vi "SparkMAXCommandPower.vi"(0 "Device Reference (in)":T2, 5 "Output Mode":T1(ring), 7 "Control Mode":enum16{"Safety", "Power"}(ring), 9 "Power or Testing Power":dbl, 11 "Error (in)":errorcluster) -> ()   [LabVIEW 2023]
doc: "Wrapper for commanding the power of a Talon FX motor controller. Supports voltage and safety interlock. Also supports the standard actuator testing interface and and the only sending new values on change."
uses:
  <vilib>/Rock Robotics/WPI/MotorControl/WPI_MotorControlDeviceRef.ctl
  <vilib>/Rock Robotics/WPI/MotorControl/WPI_MotorControlType.ctl
  <vilib>/Rock Robotics/SystemInterfaces/DIO/FPGA_DIOPWMChannel.ctl
  <vilib>/Rock Robotics/WPI/PWM/WPI_PWMDeadband.ctl
  <vilib>/Rock Robotics/SystemInterfaces/DIO/FPGA_DIOChannel.ctl
  <vilib>/Rock Robotics/WPI/ThirdParty/REV Robotics/REVLib/Typedef/Spark MAX Control Type.ctl
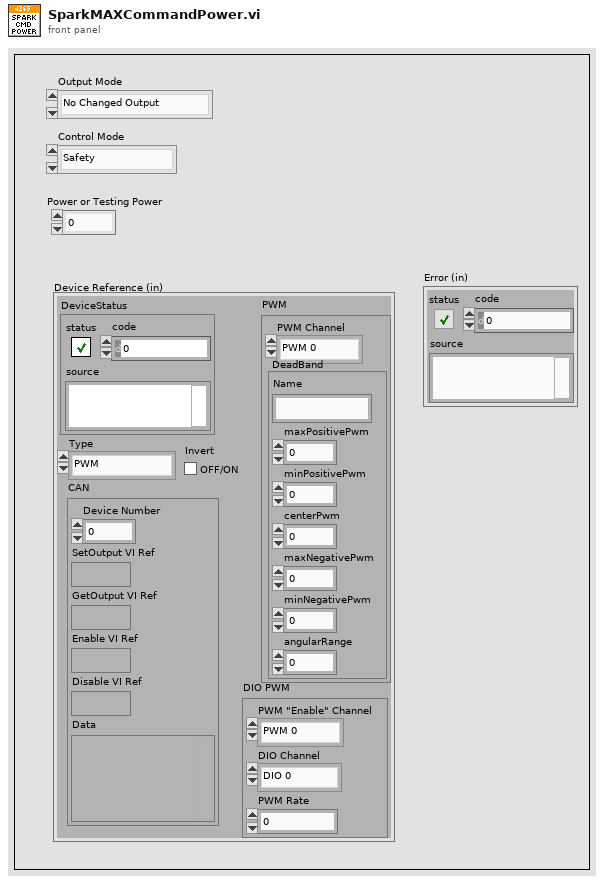
[diagram p1: front panel]
types:
  T1 = enum16{"No Changed Output", "New Normal Output", "New Testing Output"}
  T2 = typedef "WPI_MotorControlDeviceRef.ctl" = cluster{"DeviceStatus":errorcluster, "Type":T3, "PWM":cluster{"PWM Channel":T4, "DeadBand":T5}, "CAN":cluster{"Device Number":u8, "SetOutput VI Ref":variant, "GetOutput VI Ref":variant, "Enable VI Ref":variant, "Disable VI Ref":variant, "Data":variant}, "Invert":bool, "DIO PWM":cluster{"PWM \"Enable\" Channel":T4, "DIOChannel":T6, "PWM Rate":dbl}}
  T3 = typedef "WPI_MotorControlType.ctl" = enum16{"PWM", "CAN", "DIO PWM"}
  T4 = typedef "FPGA_DIOPWMChannel.ctl" = enum8{"PWM 0", "PWM 1", "PWM 2", "PWM 3", "PWM 4", "PWM 5", "PWM 6", "PWM 7", "PWM 8", "PWM 9", "PWM MXP 0", "PWM MXP 1", "PWM MXP 2", "PWM MXP 3", "PWM MXP 4", "PWM MXP 5", "PWM MXP 6", "PWM MXP 7", "PWM MXP 8", "PWM MXP 9", "Invalid"}
  T5 = typedef "WPI_PWMDeadband.ctl" = cluster{"Name":string, "maxPositivePwm":i32, "minPositivePwm":i32, "centerPwm":i32, "maxNegativePwm":i32, "minNegativePwm":i32, "angularRange":u16}
  T6 = typedef "FPGA_DIOChannel.ctl" = enum8{"DIO 0", "DIO 1", "DIO 2", "DIO 3", "DIO 4", "DIO 5", "DIO 6", "DIO 7", "DIO 8", "DIO 9", "DIO MXP 0", "DIO MXP 1", "DIO MXP 2", "DIO MXP 3", "DIO MXP 4", "DIO MXP 5", "DIO MXP 6", "DIO MXP 7", "DIO MXP 8", "DIO MXP 9", "DIO MXP 10", "DIO MXP 11", "DIO MXP 12", "DIO MXP 13", "DIO MXP 14", "DIO MXP 15", "SPI Port CS1", "SPI Port CS2", "SPI Port CS3", "SPI Port MISO", "SPI Port MOSI", "Invalid"}
  T7 = typedef "Spark MAX Control Type.ctl" = enum16{"Percent VBus", "Voltage", "Velocity", "Position", "Smart Motion", "Current", "Smart Velocity"}
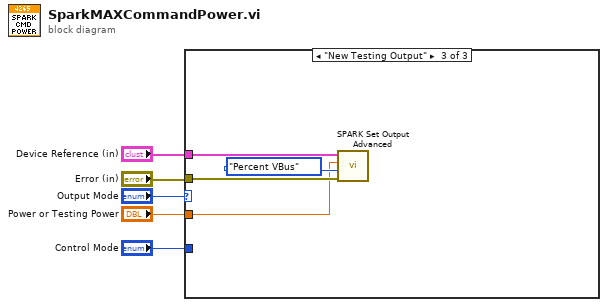
[diagram p0: block diagram]
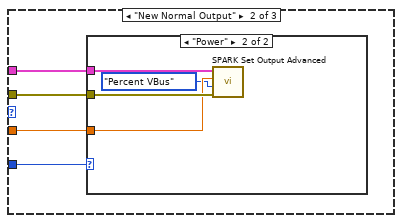
[diagram p3: hidden frame]
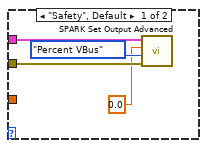
[diagram p4: hidden frame]
diagram:
  n1 = case shown="\"New Testing Output\"" "Output Mode" {
    tunnel: "Power or Testing Power" -> [_ w6 w18]
    tunnel: "Device Reference (in)" -> [_ w9 w20]
    tunnel: "Control Mode" -> [_ w8 _]
    tunnel: "Error (in)" -> [_ w7 w19]
    frame "No Changed Output", Default {
    }
    frame "New Normal Output" {
      n2 = case shown="\"Power\"" w8 {
        tunnel: w9 -> [w12 w17]
        tunnel: w6 -> [_ w15]
        tunnel: w7 -> [w11 w16]
        frame "Safety", Default {
          n3 = call <vilib>:"SPARK Set Output Advanced.vi"("error in (no error)"=w11, "Control Mode"=Spark_MAX_Control_Type."Percent VBus", "Setpoint"=0.0 ("Output"), "MotorControlDevRef"=w12) -> ()  [unwired: 6 in, 2 out]
        }
        frame "Power" {
          n4 = call <vilib>:"SPARK Set Output Advanced.vi"("error in (no error)"=w16, "Control Mode"=Spark_MAX_Control_Type."Percent VBus", "Setpoint"=w15, "MotorControlDevRef"=w17) -> ()  [unwired: 6 in, 2 out]
        }
      }
    }
    frame "New Testing Output" {
      n5 = call <vilib>:"SPARK Set Output Advanced.vi"("error in (no error)"=w19, "Control Mode"=Spark_MAX_Control_Type."Percent VBus", "Setpoint"=w18, "MotorControlDevRef"=w20) -> ()  [unwired: 6 in, 2 out]
    }
  }
